vi "OPC_UA_Disconnect_and_Stop.vi"(8 "error in (no error)":errorcluster, 10 "Refnum in":T1) -> (0 "error out":errorcluster)   [LabVIEW 2025]
uses:
  <vilib>/OPCUA/NI OPC UA Server.lvlib
  <vilib>/OPCUA/controls/OPC UA Server Refnum.ctl
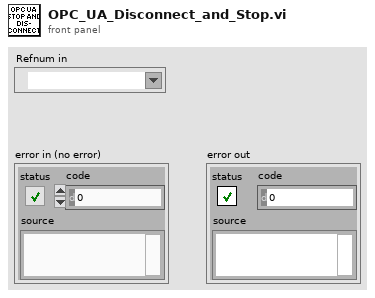
[diagram p1: front panel]
types:
  T1 = typedef "OPC UA Server Refnum.ctl" = refnum<k21>
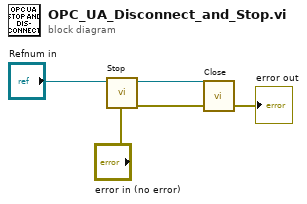
[diagram p0: block diagram]
diagram:
  n1 = call <vilib>:"Stop.vi"("error in (no error)"="error in (no error)", "OPC UA server refnum in"="Refnum in") -> ("error out"=w2:errorcluster, "OPC UA server refnum out"=w1:T1)  [unwired: 8 in]
  n2 = call <vilib>:"Close.vi"("error in (no error)"=w2, "OPC UA server refnum in"=w1) -> ("error out"=→"error out":errorcluster)  [unwired: 9 in]
